vi "CreateChan-V2.vi"(0 "Dynamic FPGA Ref":T3, 1 "Channel Config":T2(array[cluster])=[{"Channel Name"="Mod1/a0", "Sensitivity mV_EU"=1000.0, "EU"="V", "dB Ref EU"=1.0}, {"Channel Name"="Mod1/a1", "Sensitivity mV_EU"=1000.0, "EU"="V", "dB Ref EU"=1.0}, {"Channel Name"="Mod1/a2", "Sensitivity mV_EU"=1000.0, "EU"="V", "dB Ref EU"=1.0}, {"Channel Name"="Mod1/a3", "Sensitivity mV_EU"=1000.0, "EU"="V", "dB Ref EU"=1.0}, {"Channel Name"="Mod2/a0", "Sensitivity mV_EU"=1000.0, "EU"="V", "dB Ref EU"=1.0}, {"Channel Name"="Mod2/a1", "Sensitivity mV_EU"=1000.0, "EU"="V", "dB Ref EU"=1.0}, {"Channel Name"="Mod2/a2", "Sensitivity mV_EU"=1000.0, "EU"="V", "dB Ref EU"=1.0}, {"Channel Name"="Mod2/a3", "Sensitivity mV_EU"=1000.0, "EU"="V", "dB Ref EU"=1.0}, {"Channel Name"="Mod3/a0", "Sensitivity mV_EU"=1000.0, "EU"="V", "dB Ref EU"=1.0}, {"Channel Name"="Mod3/a1", "Sensitivity mV_EU"=1000.0, "EU"="V", "dB Ref EU"=1.0}, {"Channel Name"="Mod3/a2", "Sensitivity mV_EU"=1000.0, "EU"="V", "dB Ref EU"=1.0}, {"Channel Name"="Mod3/a3", "Sensitivity mV_EU"=1000.0, "EU"="V", "dB Ref EU"=1.0}, {"Channel Name"="Mod4/a0", "Sensitivity mV_EU"=1000.0, "EU"="V", "dB Ref EU"=1.0}, {"Channel Name"="Mod4/a1", "Sensitivity mV_EU"=1000.0, "EU"="V", "dB Ref EU"=1.0}, {"Channel Name"="Mod4/a2", "Sensitivity mV_EU"=1000.0, "EU"="V", "dB Ref EU"=1.0}, {"Channel Name"="Mod4/a3", "Sensitivity mV_EU"=1000.0, "EU"="V", "dB Ref EU"=1.0}, {"Channel Name"="Mod5/a0", "Sensitivity mV_EU"=1000.0, "EU"="V", "dB Ref EU"=1.0}, {"Channel Name"="Mod5/a1", "Sensitivity mV_EU"=1000.0, "EU"="V", "dB Ref EU"=1.0}, {"Channel Name"="Mod5/a2", "Sensitivity mV_EU"=1000.0, "EU"="V", "dB Ref EU"=1.0}, {"Channel Name"="Mod5/a3", "Sensitivity mV_EU"=1000.0, "EU"="V", "dB Ref EU"=1.0}, {"Channel Name"="Mod6/a0", "Sensitivity mV_EU"=1000.0, "EU"="V", "dB Ref EU"=1.0}, {"Channel Name"="Mod6/a1", "Sensitivity mV_EU"=1000.0, "EU"="V", "dB Ref EU"=1.0}, {"Channel Name"="Mod6/a2", "Sensitivity mV_EU"=1000.0, "EU"="V", "dB Ref EU"=1.0}, {"Channel Name"="Mod6/a3", "Sensitivity mV_EU"=1000.0, "EU"="V", "dB Ref EU"=1.0}] caption="Channel Name      Scale [mV/EU]              EU                           dB Ref [EU]", 2 "Configuration Sensor":T1[](array[typedef]) items=["AC Coupled", "DC Coupled", "IEPE AC Coupled"], 3 "error in":errorcluster) -> (7 "Dynamic FPGA Ref Out":T3, 8 "Sampling Info":T4, 10 "error out":errorcluster)   [LabVIEW 2015]
doc: "This VI collects and sends scaling coefficients as well as channel count to the FPGA. The number of elements in \"Channel Info\" must equal the number of channels acquired by the FPGA."
uses:
  <vilib>/NI/cRIO Wfm/SamplingInfo.ctl
  <vilib>/NI/cRIO Wfm/DynamicFPGAref.ctl
  <vilib>/LabVIEW Targets/FPGA/cRIO/shared/nicrio_ModuleControls/nicrio_cRIO-9234_ConfigModeRing.ctl
  <vilib>/rvi/errors/niLvFpgaAdjustHostInterfaceError.vi
  <vilib>/Utility/error.llb/Error Cluster From Error Code.vi
  <vilib>/rvi/interface/nirviReadWriteControl/nirviReadWriteControl.xnode
  <vilib>/NI/cRIO Wfm/cRIO Wfm.lvlib
  <vilib>/rvi/interface/Simulation/niFpgaSimulationCallBeginRW.vi
  NiFpgaLv.dll
panel:
  out "size(s)":i32
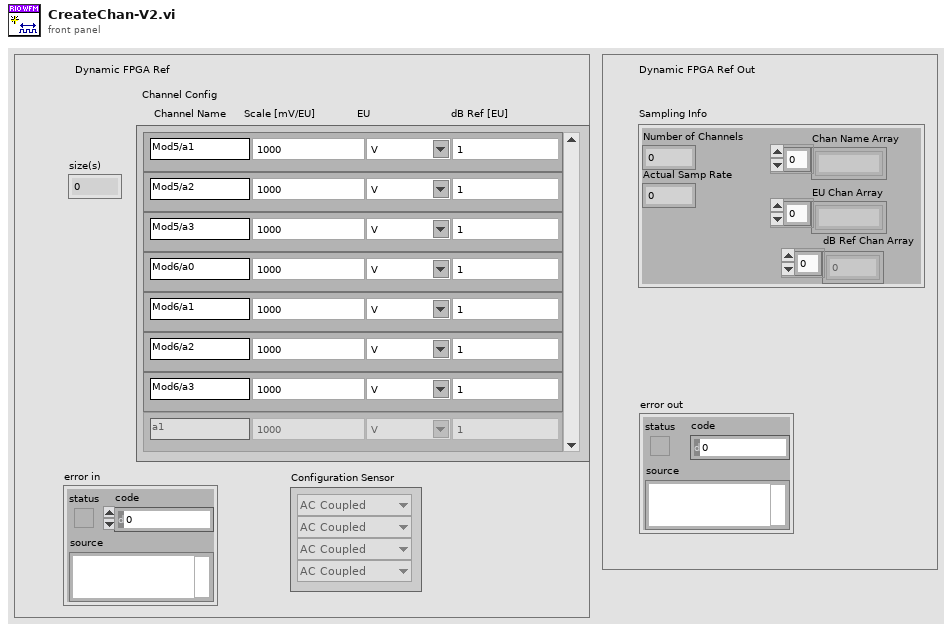
[diagram p1: front panel]
types:
  T1 = typedef "nicrio_cRIO-9234_ConfigModeRing.ctl" = u8
  T2 = cluster{"Channel Name":string, "Sensitivity mV_EU":dbl, "EU":string, "dB Ref EU":dbl}[]
  T3 = typedef "cRIO Wfm.lvlib/DynamicFPGAref.ctl" = refnum<k20>
  T4 = typedef "cRIO Wfm.lvlib/SamplingInfo.ctl" = cluster{"Number of Channels":i32, "Actual Samp Rate":dbl, "Chan Name Array":string[], "EU Chan Array":string[], "dB Ref Chan Array":dbl[]}
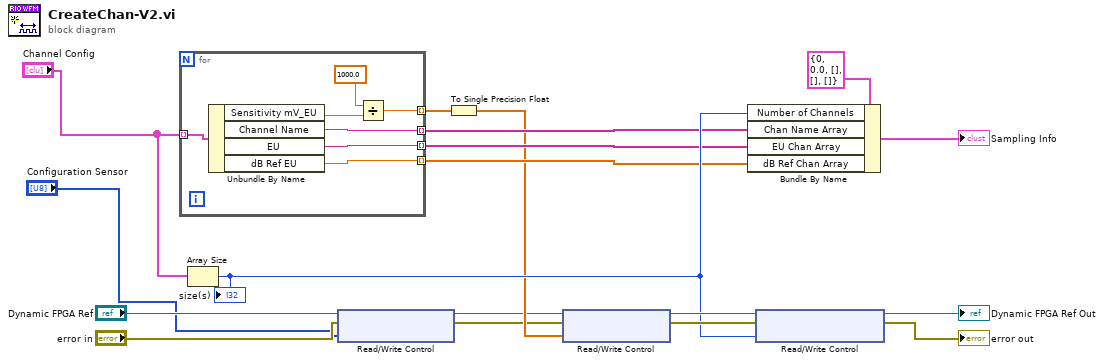
[diagram p0: block diagram]
diagram:
  n1 = for {
    tunnel: [w22] -> w11 mode=indexing
    tunnel: [w23] -> w12 mode=indexing
    tunnel: [w21] -> w10 mode=indexing
    tunnel: [w20] -> w8 mode=indexing
    tunnel: "Channel Config" -> [w19] mode=indexing
    n2 = Unbundle By Name(w19) -> ("Sensitivity mV_EU"=w24:dbl, "Channel Name"=w21:string, "EU"=w22:string, "dB Ref EU"=w23:dbl)
    n3 = Divide(x=1000.0 ("y"), y=w24) -> (x/y=w20:dbl)
  }
  n4 = Array Size(array="Channel Config") -> (size(s)=w13:i32)
  "size(s)" <- w13
  n5 = xnode "Read/Write Control"("FPGA VI Reference In"="Dynamic FPGA Ref", "error in"="error in", "Array Input Config"="Configuration Sensor") -> ("FPGA VI Reference Out"=w4:T3, "error out"=w3:errorcluster)
  n6 = To Single Precision Float(number=w8) -> (single precision float=w7:sgl[])
  n7 = xnode "Read/Write Control"("FPGA VI Reference In"=w4, "error in"=w3, "Chan Scale Array"=w7) -> ("FPGA VI Reference Out"=w15:T3, "error out"=w14:errorcluster)
  n8 = Bundle By Name(cluster=T4 {"Number of Channels"=0, "Actual Samp Rate"=0.0, "Chan Name Array"=[], "EU Chan Array"=[], "dB Ref Chan Array"=[]} ("Sampling Info"), "Number of Channels"=w13, "Chan Name Array"=w10, "EU Chan Array"=w11, "dB Ref Chan Array"=w12) -> (→"Sampling Info":T4)
  n9 = xnode "Read/Write Control"("FPGA VI Reference In"=w15, "error in"=w14, "Number of Channels"=w13) -> ("FPGA VI Reference Out"=→"Dynamic FPGA Ref Out":T3, "error out"=→"error out":errorcluster)
